vi "error_window.vi"(7 "callee":refnum<vi>, 8 "error in (no error)":errorcluster, 10 "configuration":T3, 11 "v1 in":refnum<class "v1.lvclass">) -> (0 "error out":errorcluster, 2 "dialog_selection":T4=enum."button_2", 3 "v1 out":refnum<class "v1.lvclass">)   [LabVIEW 2015, in "lv-dialog.lvlib" / "v1.lvlib" / "v1.lvclass"]
doc: "The error window is meant to approximate the simple error handler. The implementation is kind of jank/garbage, but it's functional.\n\nThis IS implemented by the base api class using the \"General Error Handler.vi\""
uses:
  v1.lvclass
  _controls/selection.ctl
  <vilib>/Utility/error.llb/DialogTypeEnum.ctl
  <vilib>/Utility/error.llb/TagReturnType.ctl
  v1.lvlib
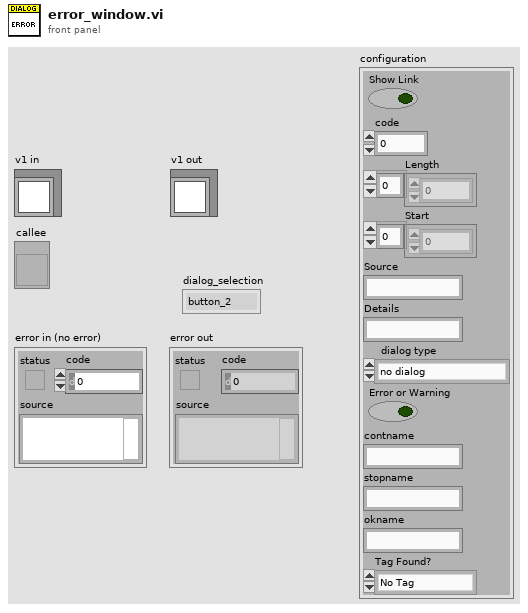
[diagram p1: front panel]
types:
  T1 = typedef "DialogTypeEnum.ctl" = enum16{"no dialog", "OK message", "continue or stop message", "auto error handling dialog", "OK message + warnings", "continue/stop + warnings"}
  T2 = typedef "TagReturnType.ctl" = enum16{"No Tag", "<err>", "<append>"}
  T3 = cluster{"Show Link":bool, "code":i32, "Length":i32[], "Start":i32[], "Source":string, "Details":string, "dialog type":T1, "Error or Warning":bool, "contname":string, "stopname":string, "okname":string, "Tag Found?":T2}
  T4 = typedef "lv-dialog.lvlib/v1.lvlib/selection.ctl" = enum16{"null", "panel_closed", "button_1", "button_2", "button_3", "cancelled"}
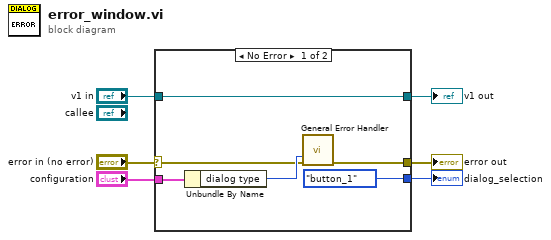
[diagram p0: block diagram]
diagram:
  n1 = case shown="No Error" "error in (no error)" {
    selector: "error in (no error)" -> [w9 w14]
    tunnel: [w8 w14] -> w5
    tunnel: [w12 w13] -> w3
    tunnel: "v1 in" -> [w12 w13]
    tunnel: "configuration" -> [w11 _]
    tunnel: [selection."button_1" ("dialog_selection") _] -> w1
    frame No Error {
      n2 = Unbundle By Name(w11) -> ("dialog type"=w10:T1)
      n3 = call <vilib>:"General Error Handler.vi"("type of dialog (OK msg:1)"=w10, "error in (no error)"=w9) -> ("error out"=w8:errorcluster)  [unwired: 9 in, 4 out]
    }
    frame Error {
    }
  }
  "error out" <- w5
  "v1 out" <- w3
  "dialog_selection" <- w1
